vi "23-lsync.vi"(3 "this":i32, 4 "Count in":i32, 5 "button":i32, 6 "Cluster":T1={"Auto1"=TRUE, "Auto2"=TRUE, "Rel1"=FALSE, "Rel2"=FALSE, "Filt1"=FALSE, "Filt2"=FALSE, "Rate"=enum."Slow", "Range1"=enum."10mV", "Range2"=enum."100mV", "Filt3"=FALSE, "Filt4"=FALSE, "Rel temp 1"=FALSE, "Analog1"=FALSE, "Analog2"=FALSE, "Analog temp 1"=FALSE, "Digital1"=FALSE, "Digital2"=FALSE, "Digital temp 1 "=FALSE, "Window1"=enum."None", "Window2"=enum."None", "Window temp 1"=enum."None", "RDGS1"="010", "RDGS2"="010", "RDGS temp 1"="010", "Type_type1"=TRUE, "Type_type2"=TRUE, "Type_type temp 1"=TRUE, "LSync"=FALSE, "Unit"=enum."C", "Sens"=TRUE, "Type tcoupl"=enum."J", "Junc"=TRUE, "prevState"=0, "Rel temp 2"=FALSE, "Analog temp 2"=FALSE, "Digital temp 2"=FALSE, "Type_type temp 2"=TRUE, "RDGS temp 2"="010", "Window temp 2"=enum."None", "address"="0"}) -> (0 "next state":i32, 1 "Count out":i32, 2 "Cluster 2":T1)   [LabVIEW 2017]
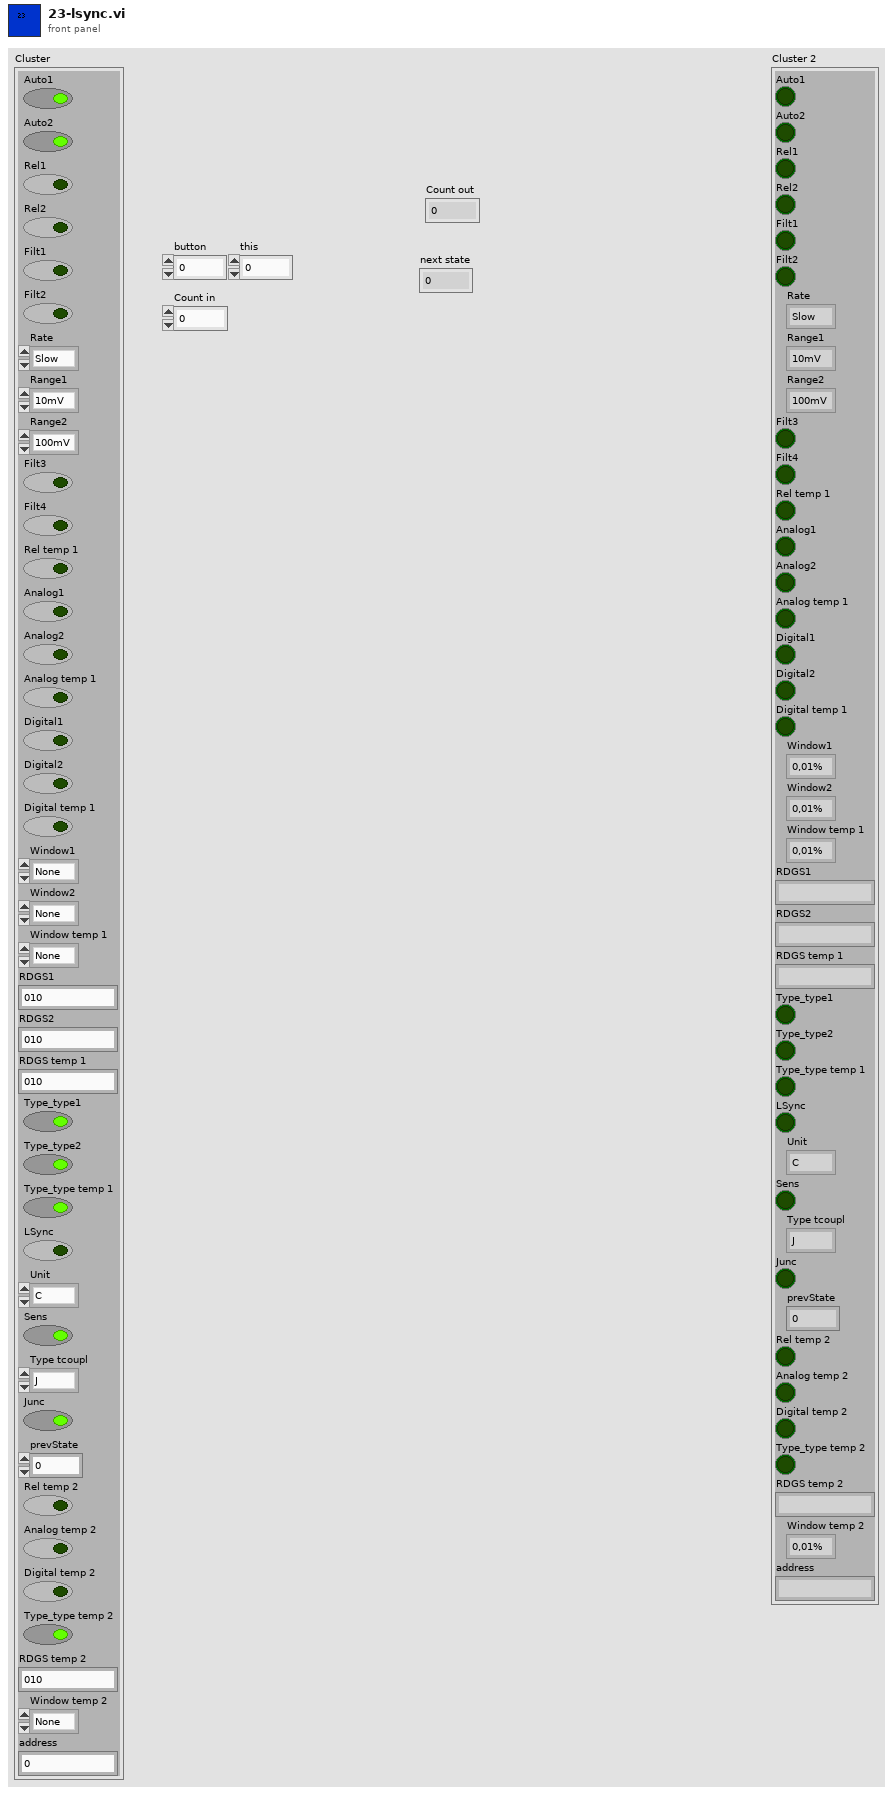
[diagram p1: front panel]
types:
  T1 = cluster{"Auto1":bool, "Auto2":bool, "Rel1":bool, "Rel2":bool, "Filt1":bool, "Filt2":bool, "Rate":enum16{"Slow", "Fast", "Med"}, "Range1":enum16{"10mV", "100mV", "1V", "10V", "100V"}, "Range2":enum16{"100mV", "1V", "10V"}, "Filt3":bool, "Filt4":bool, "Rel temp 1":bool, "Analog1":bool, "Analog2":bool, "Analog temp 1":bool, "Digital1":bool, "Digital2":bool, "Digital temp 1 ":bool, "Window1":enum16{"0,01%", "0,1%", "1%", "10%", "None"}, "Window2":enum16{"0,01%", "0,1%", "1%", "10%", "None"}, "Window temp 1":enum16{"0,01%", "0,1%", "1%", "10%", "None"}, "RDGS1":string, "RDGS2":string, "RDGS temp 1":string, "Type_type1":bool, "Type_type2":bool, "Type_type temp 1":bool, "LSync":bool, "Unit":enum16{"C", "K", "F"}, "Sens":bool, "Type tcoupl":enum16{"J", "K", "T", "E", "R", "S", "B", "N"}, "Junc":bool, "prevState":i32, "Rel temp 2":bool, "Analog temp 2":bool, "Digital temp 2":bool, "Type_type temp 2":bool, "RDGS temp 2":string, "Window temp 2":enum16{"0,01%", "0,1%", "1%", "10%", "None"}, "address":string}
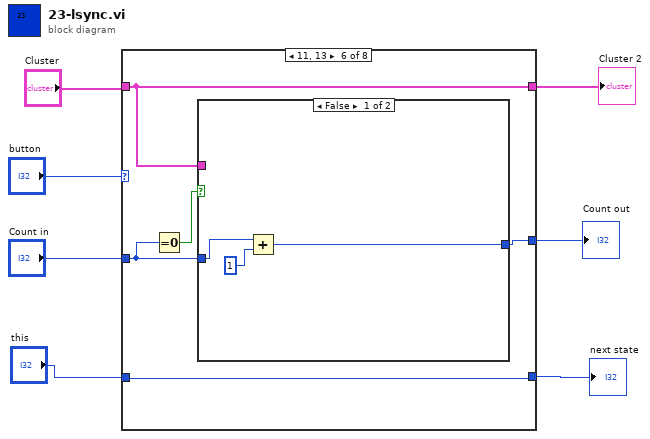
[diagram p0: block diagram]
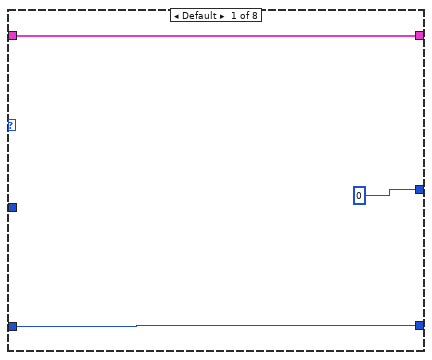
[diagram p2: hidden frame]
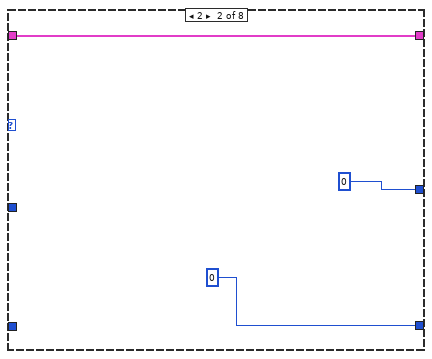
[diagram p3: hidden frame]
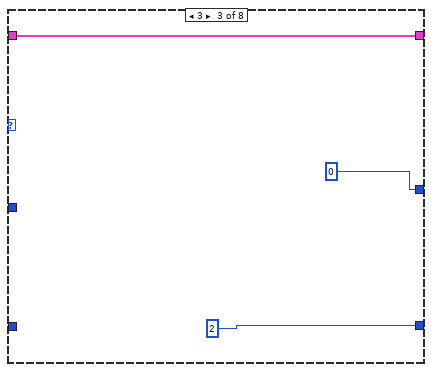
[diagram p4: hidden frame]
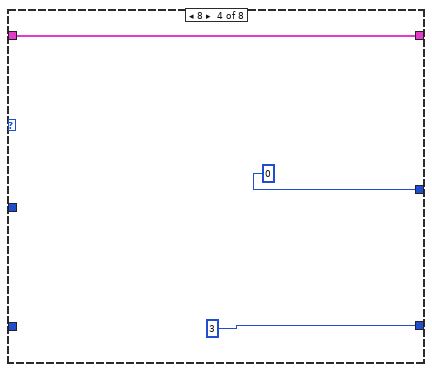
[diagram p5: hidden frame]
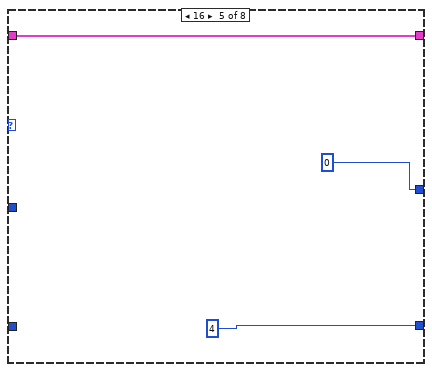
[diagram p6: hidden frame]
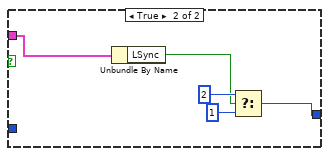
[diagram p7: hidden frame]
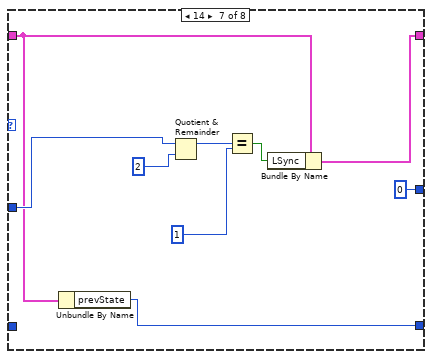
[diagram p8: hidden frame]
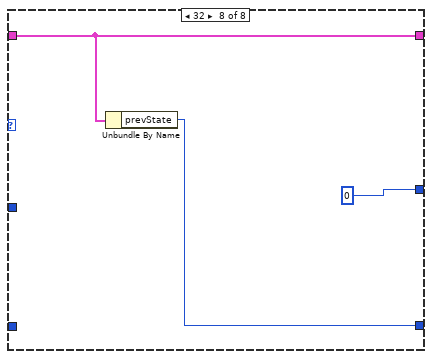
[diagram p9: hidden frame]
diagram:
  n1 = case shown="11, 13" "button" {
    tunnel: [w9 0 ("this") 2 3 4 w27 w36 w46] -> w4
    tunnel: "this" -> [w9 _ _ _ _ w27 _ _]
    tunnel: "Cluster" -> [w10 w13 w15 w18 w21 w25 w41 w47]
    tunnel: [w10 w13 w15 w18 w21 w25 w44 w47] -> w5
    tunnel: "Count in" -> [_ _ _ _ _ w23 w43 _]
    tunnel: [0 ("t") 0 ("t") 0 ("t") 0 ("t") 0 ("t") w26 0 ("t") 0 ("t")] -> w2
    frame Default {
    }
    frame 2 {
    }
    frame 3 {
    }
    frame 8 {
    }
    frame 16 {
    }
    frame 11, 13 {
      n2 = Equal To 0?(x=w23) -> (x = 0?=w24:bool)
      n3 = case shown="False" w24 {
        tunnel: [w29 w35] -> w26
        tunnel: w25 -> [_ w34]
        tunnel: w23 -> [w28 _]
        frame False {
          n4 = Add(x=w28, y=1) -> (x+y=w29:i32)
        }
        frame True {
          n5 = Unbundle By Name(w34) -> ("LSync"=w31:bool)
          n6 = Select(t=2, s=w31, f=1) -> (s? t:f=w35:i32)
        }
      }
    }
    frame 14 {
      n7 = Unbundle By Name(w41) -> ("prevState"=w36:i32)
      n8 = Quotient & Remainder(x=w43, y=2) -> (x-y*floor(x/y)=w38:i32)  [unwired: 1 out]
      n9 = Equal?(x=w38, y=1 ("x")) -> (x = y?=w39:bool)
      n10 = Bundle By Name(cluster=w41, "LSync"=w39) -> (w44:T1)
    }
    frame 32 {
      n11 = Unbundle By Name(w47) -> ("prevState"=w46:i32)
    }
  }
  "next state" <- w4
  "Count out" <- w2
  "Cluster 2" <- w5
